vi "IMAQ Testing.vi"() -> ()   [LabVIEW 2011]
uses:
  <vilib>/Platform/TimedLoop/XDataNode/timing_clust.ctl
  <vilib>/Platform/TimedLoop/XDataNode/nitl_modes.ctl
  <vilib>/Platform/TimedLoop/XDataNode/wakeup.ctl
  <vilib>/Platform/TimedLoop/XDataNode/XDataNode.xnode
  <vilib>/Platform/TimedLoop/XDataNode/XDNodeRunTimeDep.lvlib
panel:
  in  "element":i16
  in  "stop":bool
  out "Image":T1(plugin-control)
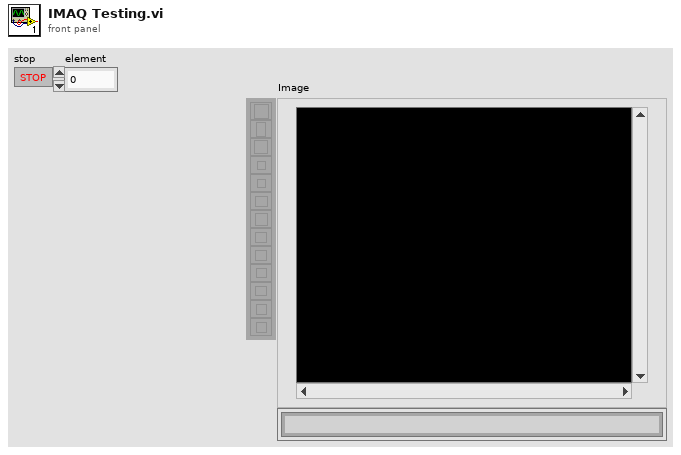
[diagram p1: front panel]
types:
  T1 = typedef "IMAQ Image.ctl" = refnum<image>
  T2 = typedef "XDNodeRunTimeDep.lvlib/timing_clust.ctl" = cluster{"Expected End [f-1]":u64, "Actual End [f-1]":u64, "Finished Late? [f-1]":bool, "Expected End [i-1]":u64, "Actual End [i-1]":u64, "Finished Late? [i-1]":bool, "Expected Start [i]":u64, "Actual Start [i]":u64, "Expected Start [f]":u64, "Actual Start [f]":u64, "Source Name":string, "Structure Name":string, "Period":i64, "Deadline":i64, "Offset":i64, "Start":i64, "Priority":i32, "Timeout":i32, "Mode":T3, "Wakeup Reason":T4, "Error":errorcluster, "Source Type":string, "Secondary Source Type":string, "Global End Time":u64, "Global Start Time":u64, "Frame Duration":u64, "Iteration Duration":u64, "Assigned CPU":i32, "I/O Scan Engine Mode":u32}
  T3 = typedef "XDNodeRunTimeDep.lvlib/nitl_modes.ctl" = enum32{"No Change", "Process missed periods, maintain original phase", "Discard missed periods, maintain original phase", "Process missed periods, ignore original phase", "Discard missed periods, ignore original phase"}
  T4 = typedef "XDNodeRunTimeDep.lvlib/wakeup.ctl" = enum32{"Normal", "Aborted", "Asynchronous wakeup", "Timing source error", "Timed loop error", "Timeout"}
  T5 = typedef "Image Type" = u32
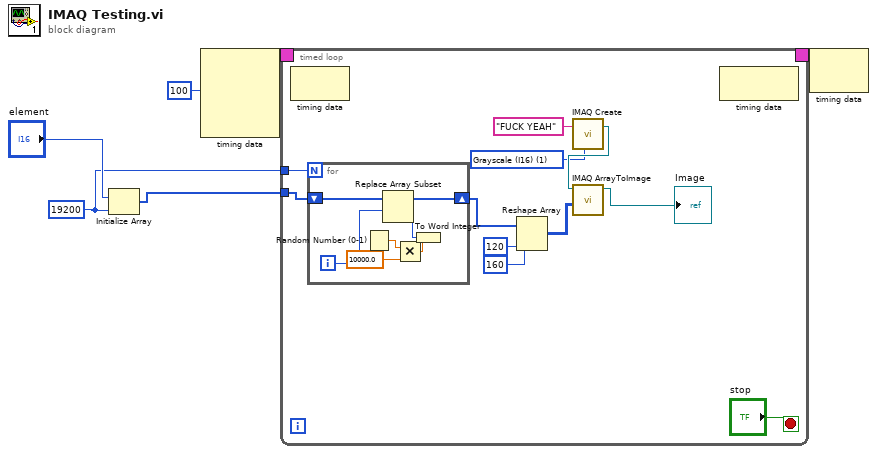
[diagram p0: block diagram]
diagram:
  w2 = 19200 ("dimension size")
  n1 = Initialize Array("element", w2) -> (w3:i16[])
  n2 = node-c288(i64 100 ("Period")) -> (w5:T2)  [unwired: 3 in]
  n3 = timed-loop {
    timing: w5 -> [_]
    timing-out: [_] -> w4
    tunnel: w3 -> [w12]
    tunnel: w2 -> [w7]
    stop <- "stop" stop-if-true
    w14 = T5 1 items=["Grayscale (U8)", "Grayscale (I16)", "Grayscale (SGL)", "Complex (CSG)", "RGB (U32)", "HSL (U32)", "RGB (U64)", "Grayscale (U16)"] ("Image Type")
    n4 = node-c288() -> ()  [unwired: 1 in, 1 out]
    n5 = for {
      N: w7 -> [_]
      shift-right: [w26] -> w9
      shift-left: w12 -> [w24]
      i -> [w25]
      n6 = Random Number (0-1)() -> (number: 0 to 1=w23:dbl)
      n7 = Multiply(x=w23, y=10000.0) -> (x*y=w21:dbl)
      n8 = To Word Integer(number=w21) -> (16bit integer=w20:i16)
      n9 = Replace Array Subset(array=w24, new element=w20, index=w25) -> (w26:i16[])
    }
    n10 = Reshape Array(w9, 120 ("dimension size"), 160 ("dimension size")) -> (w8:i16[][])
    n11 = call "IMAQ Create"("Image Name"="FUCK YEAH", "Image Type"=w14) -> ("New Image"=w17:T1)  [unwired: 3 in, 1 out]
    n12 = call "IMAQ ArrayToImage"("Image Pixels (I16)"=w8, "Image"=w17) -> ("Image Out"=→"Image":T1)  [unwired: 8 in, 1 out]
    n13 = node-c288() -> ()  [unwired: 1 in, 1 out]
  }
  n14 = node-c288(w4) -> ()  [unwired: 1 out]
